vi "Cleanup.vi"(8 "error in (no error)":errorcluster, 11 "AST in":refnum<class "AST.lvclass">) -> (0 "error out":errorcluster)   [LabVIEW 2020, in "PicoG-ParserLexer.lvlib" / "AST.lvclass"]
uses:
  AST.lvclass
  Symbol Map/Symbol Map.lvclass
  Node/Node.lvclass
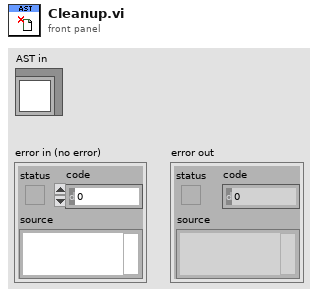
[diagram p1: front panel]
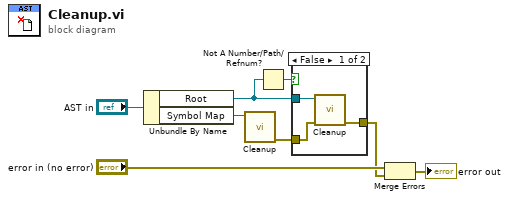
[diagram p0: block diagram]
diagram:
  n1 = Unbundle By Name("AST in") -> ("Root"=w3:refnum<data-value>, "Symbol Map"=w6:refnum<class "Symbol Map.lvclass">)
  n2 = call "Cleanup.vi"("Symbol Map in"=w6) -> ("error out"=w4:errorcluster)  [unwired: 10 in]
  n3 = Not A Number/Path/Refnum?(number/path/refnum=w3) -> (NaN/Path/Refnum?=w5:bool)
  n4 = case shown="False" w5 {
    tunnel: w4 -> [w10 w12]
    tunnel: w3 -> [w11 _]
    tunnel: [w9 w12] -> w1
    frame False {
      n5 = call "Cleanup.vi"("error in (no error)"=w10, "NodeRef In"=w11) -> ("error out"=w9:errorcluster)  [unwired: 9 in]
    }
    frame True {
    }
  }
  n6 = Merge Errors("error in (no error)", w1) -> (→"error out":errorcluster)
